vi "19-Orientations.vi"(11 "Sensor":cluster{"Name":string, "Beacons":i32[][]}) -> (3 "Orientations":T1(array[cluster]))   [LabVIEW 2019, in "19.lvlib"]
uses:
  19.lvlib
panel:
  out "XZ":cluster{"Beacons":i32[], "Beacons":i32[]}(graph)
  out "ZY":cluster{"Beacons":i32[], "Beacons":i32[]}(graph)
  out "XY":cluster{"Beacons":i32[], "Beacons":i32[]}(graph)
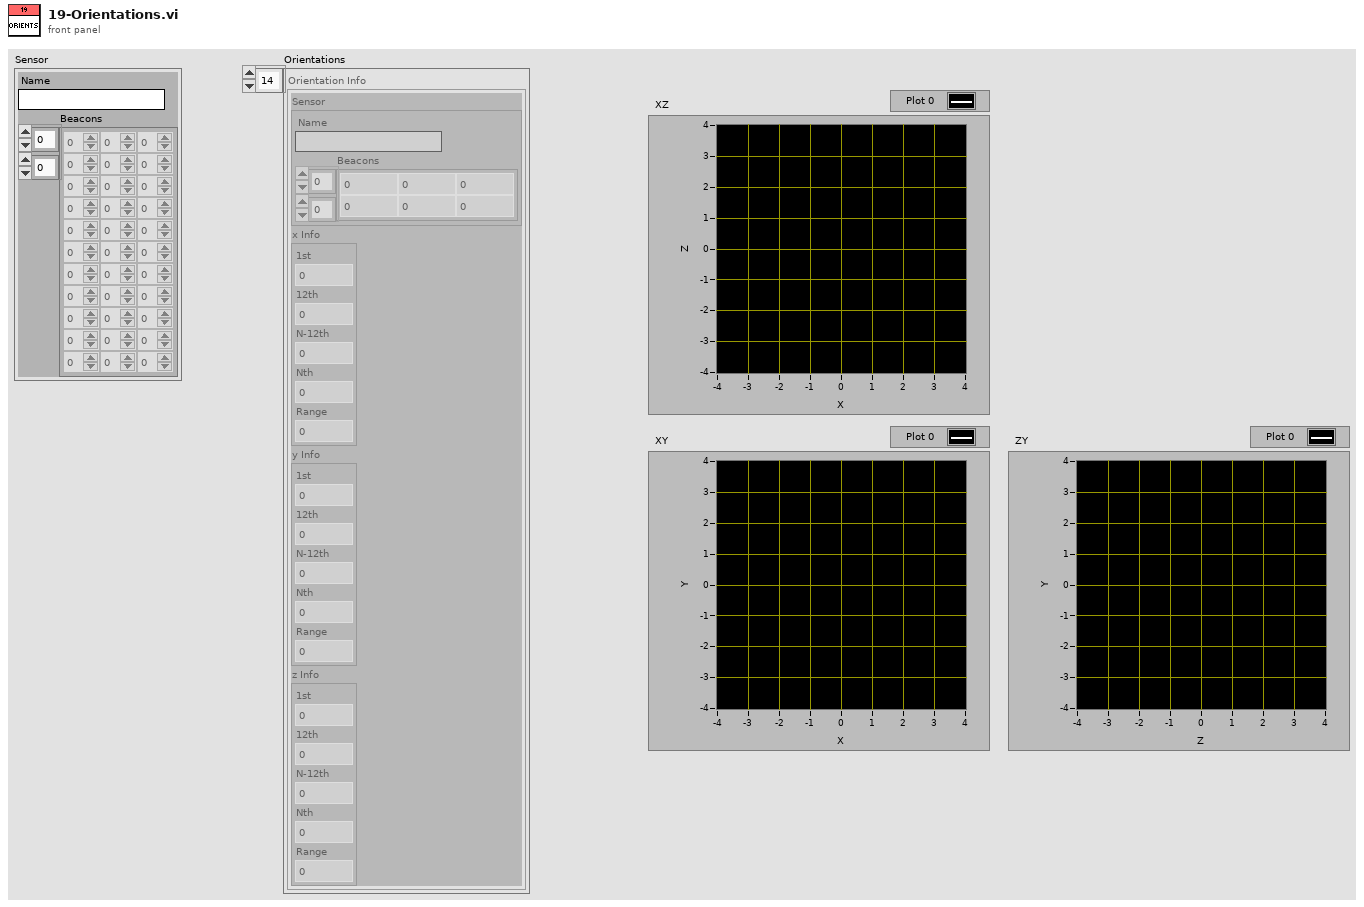
[diagram p1: front panel]
types:
  T1 = cluster{"Sensor":cluster{"Name":string, "Beacons":i32[][]}, "x Info":cluster{"1st":i32, "12th":i32, "N-12th":i32, "Nth":i32, "Range":i32}, "y Info":cluster{"1st":i32, "12th":i32, "N-12th":i32, "Nth":i32, "Range":i32}, "z Info":cluster{"1st":i32, "12th":i32, "N-12th":i32, "Nth":i32, "Range":i32}}[]
  T2 = cluster{"Sensor":cluster{"Name":string, "Beacons":i32[][]}, "x Info":cluster{"1st":i32, "12th":i32, "N-12th":i32, "Nth":i32, "Range":i32}, "y Info":cluster{"1st":i32, "12th":i32, "N-12th":i32, "Nth":i32, "Range":i32}, "z Info":cluster{"1st":i32, "12th":i32, "N-12th":i32, "Nth":i32, "Range":i32}}
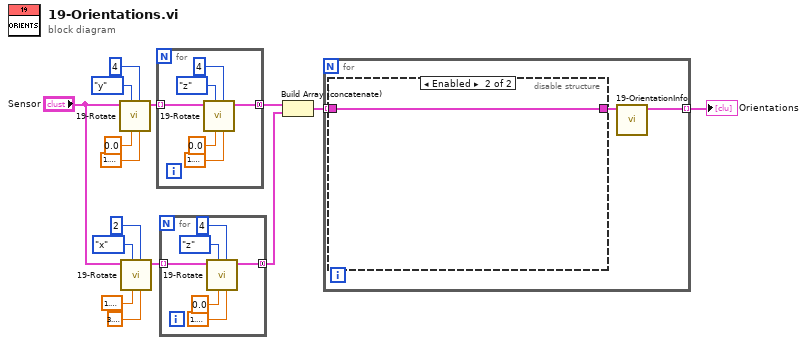
[diagram p0: block diagram]
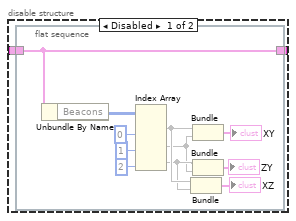
[diagram p2: hidden frame]
diagram:
  n1 = call "19-Rotate.vi"("Rotate By"=1.5707963267948966, "Number of Rotations"=4, "Initial Rotation"=0.0, "Rotation Axis"=enum16{"x", "y", "z"}."y", "Sensor"="Sensor") -> ("Sensor Rotations"=w11:cluster{"Name":string, "Beacons":i32[][]}[])  [unwired: 6 in]
  n2 = call "19-Rotate.vi"("Rotate By"=3.141592653589793, "Number of Rotations"=2, "Initial Rotation"=1.5707963267948966, "Rotation Axis"=enum16{"x", "y", "z"}."x", "Sensor"="Sensor") -> ("Sensor Rotations"=w3:cluster{"Name":string, "Beacons":i32[][]}[])  [unwired: 6 in]
  n3 = for {
    tunnel: [w16] -> w12 mode=concatenating
    tunnel: w11 -> [w17] mode=indexing
    n4 = call "19-Rotate.vi"("Rotate By"=1.5707963267948966, "Number of Rotations"=4, "Initial Rotation"=0.0, "Rotation Axis"=enum16{"x", "y", "z"}."z", "Sensor"=w17) -> ("Sensor Rotations"=w16:cluster{"Name":string, "Beacons":i32[][]}[])  [unwired: 6 in]
  }
  n5 = for {
    tunnel: [w22] -> w2 mode=concatenating
    tunnel: w3 -> [w23] mode=indexing
    n6 = call "19-Rotate.vi"("Rotate By"=1.5707963267948966, "Number of Rotations"=4, "Initial Rotation"=0.0, "Rotation Axis"=enum16{"x", "y", "z"}."z", "Sensor"=w23) -> ("Sensor Rotations"=w22:cluster{"Name":string, "Beacons":i32[][]}[])  [unwired: 6 in]
  }
  n7 = Build Array (concatenate)(w12, w2) -> (w15:cluster{"Name":string, "Beacons":i32[][]}[])
  n8 = for {
    tunnel: w15 -> [w29] mode=indexing
    tunnel: [w30] -> w14 mode=indexing
    n9 = disable-structure shown="Enabled" {
      disable-tunnel: w29 -> [w32 w44]
      disable-tunnel: [w31 w44] -> w28
      frame Disabled {
        n10 = flat-sequence {
          tunnel: w32 -> [w35]
          tunnel: [w35] -> _
          tunnel: [w35] -> w31
          frame #0 {
            n11 = Unbundle By Name(w35) -> ("Beacons"=w43:i32[][])
            n12 = Index Array(array=w43, index (col) #1=0 ("disabled index (col)"), index (col) #2=1 ("index (col)"), index (col) #3=2 ("index (col)")) -> (element #1=w39:i32[], element #2=w33:i32[], element #3=w34:i32[])  [unwired: 3 in]
            n13 = Bundle("Beacons"=w39, "Beacons"=w34) -> (→"XZ":cluster{"Beacons":i32[], "Beacons":i32[]})  [unwired: 1 in]
            n14 = Bundle("Beacons"=w39, "Beacons"=w33) -> (→"XY":cluster{"Beacons":i32[], "Beacons":i32[]})  [unwired: 1 in]
            n15 = Bundle("Beacons"=w34, "Beacons"=w33) -> (→"ZY":cluster{"Beacons":i32[], "Beacons":i32[]})  [unwired: 1 in]
          }
        }
      }
      frame Enabled {
      }
    }
    n16 = call "19-OrientationInfo.vi"("Sensor in"=w28) -> ("Orientation Info"=w30:T2)  [unwired: 10 in]
  }
  "Orientations" <- w14
